vi "Initialize.vi"(7 "Channel Name":string="Setpoint.ch%d.SP", 8 "error in":errorcluster, 9 "Number of Channels":u32=1, 10 "Instance Name":string="PluginName", 11 "Pressure Setpoint in":refnum<class "Pressure Setpoint.lvclass">) -> (0 "error out":errorcluster, 2 "Channel":T1[](array[typedef]), 3 "Pressure Setpoint out":refnum<class "Pressure Setpoint.lvclass">)   [LabVIEW 2023, in "Pressure Setpoint.lvclass"]
uses:
  Pressure Setpoint.lvclass
  Pressure Setpoint.lvclass/Pressure Setpoint.ctl
  Parents/Setpoint/Setpoint.lvclass
  Utilities/Channel.ctl
  Utilities/Utilities.lvlib
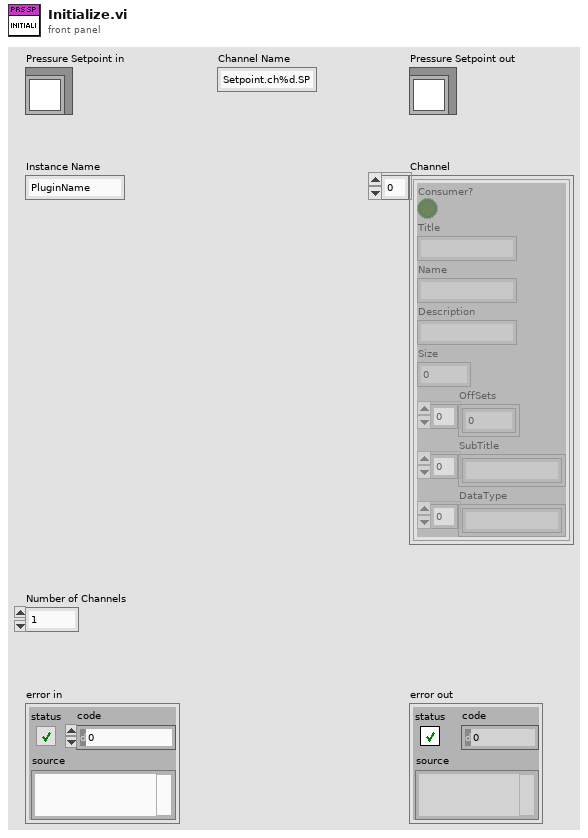
[diagram p1: front panel]
types:
  T1 = typedef "Utilities.lvlib/Channel.ctl" = cluster{"Consumer?":bool, "Title":string, "Name":string, "Description":string, "Size":i32, "OffSets":i32[], "SubTitle":string[], "DataType":string[]}
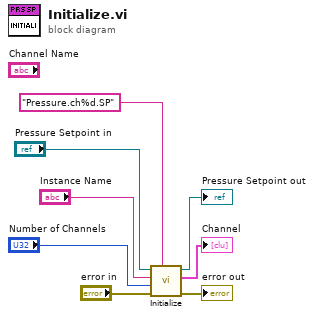
[diagram p0: block diagram]
diagram:
  n1 = call-parent "Initialize.vi"("Channel Name"="Pressure.ch%d.SP", "error in"="error in", "Number of Channels"="Number of Channels", "Instance Name"="Instance Name", "Setpoint in"="Pressure Setpoint in") -> ("error out"=→"error out":errorcluster, "Channel"=→"Channel":T1[], "Setpoint out"=→"Pressure Setpoint out":refnum<class "Pressure Setpoint.lvclass">)  [unwired: 4 in]
